vi "Close.vi"(8 "error in (no error)":errorcluster, 11 "Watchdog":refnum<data-value>) -> (0 "error out":errorcluster)   [LabVIEW 2017, in "Watchdog.lvclass"]
doc: "Close the watchdog reference."
uses:
  <vilib>/NI/Software Watchdog/Watchdog/Watchdog.lvclass
  <vilib>/NI/Software Watchdog/Watchdog/Watchdog.lvclass/Watchdog.ctl
  <vilib>/NI/Software Watchdog/Pound/Pound.lvclass
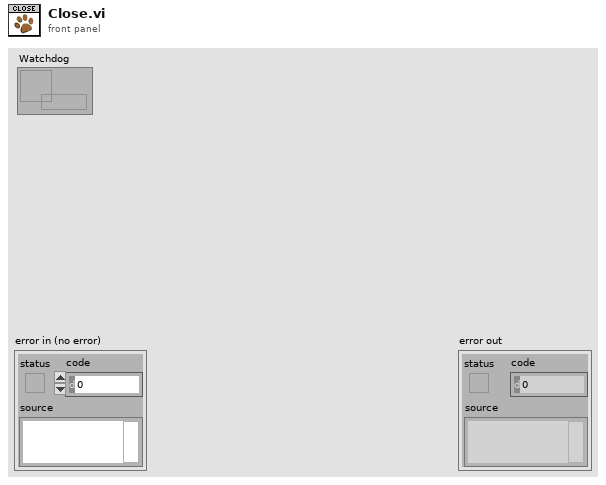
[diagram p1: front panel]
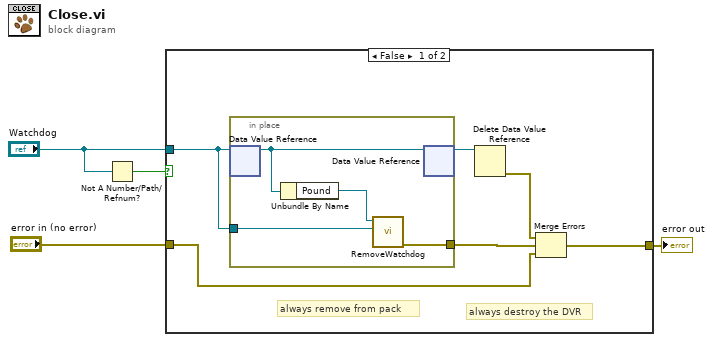
[diagram p0: block diagram]
diagram:
  n1 = Not A Number/Path/Refnum?(number/path/refnum="Watchdog") -> (NaN/Path/Refnum?=w1:bool)
  n2 = case shown="False" w1 {
    tunnel: "error in (no error)" -> [w5 w15]
    tunnel: [w6 w15] -> w3
    tunnel: "Watchdog" -> [w9 _]
    frame False {
      # "always remove from pack"
      # "always destroy the DVR"
      n3 = in-place {
        in-place-border: w9 -> [w12]
        in-place-border: [w11] -> w8
        n4 = in-place-dvr #1(w9) -> (w14:refnum<class "Watchdog.lvclass">)  [unwired: 1 out]
        n5 = Unbundle By Name(w14) -> ("Pound"=w13:refnum<class "Pound.lvclass">)
        n6 = call <vilib>:"RemoveWatchdog.vi"("Watchdog"=w12, "Pound in"=w13) -> ("error out"=w11:errorcluster)  [unwired: 8 in, 1 out]
        n7 = in-place-dvr #1(w14) -> (w10:refnum<data-value>)  [unwired: 1 out]
      }
      n8 = Delete Data Value Reference(data value reference=w10) -> (error out=w7:errorcluster)  [unwired: 1 in, 1 out]
      n9 = Merge Errors(w7, w8, w5) -> (w6:errorcluster)
    }
    frame True {
      # "watchdog has already been destroyed"
    }
  }
  "error out" <- w3
